vi "FlatToRichrfcontrol_DeviceInformationResponse.vi"(5 "OutputClusterType":T1, 11 "InputCluster":T2) -> (3 "OutputCluster":T1)   [LabVIEW 2024, in "FlexSDR_gRPC_client.lvlib"]
uses:
  FlexSDR_gRPC_client.lvlib
  rfcontrol_DeviceInformationResponse_Flat.ctl
  rfcontrol_DeviceInformationResponse.ctl
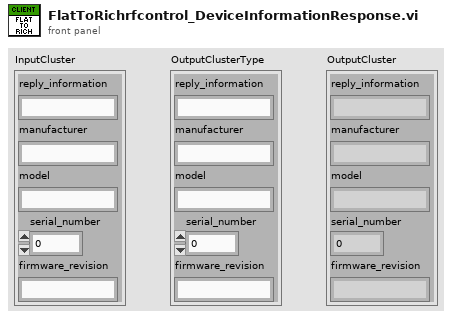
[diagram p1: front panel]
types:
  T1 = typedef "FlexSDR_gRPC_client.lvlib/rfcontrol_DeviceInformationResponse.ctl" = cluster{"reply_information":string, "manufacturer":string, "model":string, "serial_number":i32, "firmware_revision":string}
  T2 = typedef "FlexSDR_gRPC_client.lvlib/rfcontrol_DeviceInformationResponse_Flat.ctl" = cluster{"reply_information":string, "manufacturer":string, "model":string, "serial_number":i32, "firmware_revision":string}
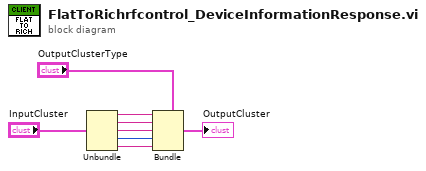
[diagram p0: block diagram]
diagram:
  n1 = Unbundle "Unbundle"("InputCluster") -> ("reply_information"=w5:string, "manufacturer"=w4:string, "model"=w3:string, "serial_number"=w2:i32, "firmware_revision"=w1:string)
  n2 = Bundle "Bundle"(cluster="OutputClusterType", "reply_information"=w5, "manufacturer"=w4, "model"=w3, "serial_number"=w2, "firmware_revision"=w1) -> (→"OutputCluster":T1)
